vi "Read Delay.vi"(8 "error in (no error)":errorcluster, 10 "milliseconds to wait":u32, 11 "Model_AMC in":refnum<class "Model_AMC.lvclass">) -> (0 "error out":errorcluster, 3 "Model_AMC out":refnum<class "Model_AMC.lvclass">)   [LabVIEW 2021, in "Model_AMC.lvclass"]
uses:
  Model_AMC.lvclass
  Model_AMC.lvclass/Model_AMC.ctl
  552c0f18-c5b7-472d-951e-eba6239c8f6f.vi
  fee96ba8-812a-446b-8deb-08a52aa84ac4.vi
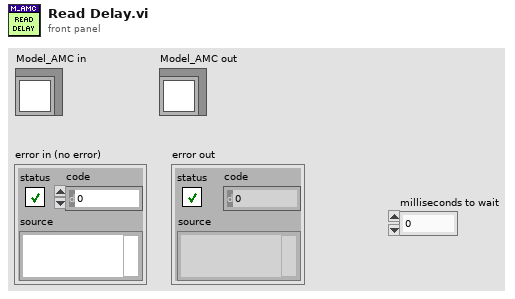
[diagram p1: front panel]
types:
  T1 = typedef "AMC_FW.lvlib/Queue.ctl" = cluster{"Q":T2, "Name":string}
  T2 = typedef "AMC_FW.lvlib/Message Queue.ctl" = refnum<queue>
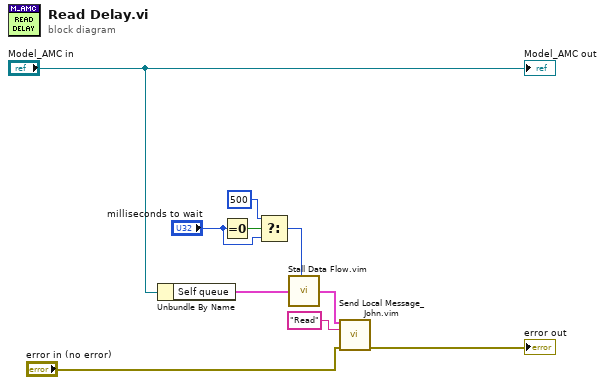
[diagram p0: block diagram]
diagram:
  n1 = Unbundle By Name("Model_AMC in") -> ("Self queue"=w7:T1)
  n2 = Equal To 0?(x="milliseconds to wait") -> (x = 0?=w9:bool)
  n3 = Select(t=u32 500 ("milliseconds to wait"), s=w9, f="milliseconds to wait") -> (s? t:f=w4:u32)
  n4 = call "Stall Data Flow.vim"("value in"=w7, "milliseconds to wait"=w4) -> ("value out"=w5:T1)  [unwired: 1 out]
  n5 = call "Send Local Message_John.vim"("Queue In"=w5, "Elements at Back"="Read", "error in"="error in (no error)") -> ("error out"=→"error out":errorcluster)  [unwired: 10 in, 2 out]
  "Model_AMC out" <- "Model_AMC in"
